vi "sq_calibrate.vi"() -> ()   [LabVIEW 2014]
uses:
  <vilib>/Analysis/6fits.llb/Curve Fitting Criteria.ctl
  <vilib>/Platform/TimedLoop/XDataNode/timing_clust.ctl
  <vilib>/Platform/TimedLoop/XDataNode/nitl_modes.ctl
  <vilib>/Platform/TimedLoop/XDataNode/wakeup.ctl
  testing/injection_point.ctl
  cancellation/decoupled_gain.ctl
  testing/probe_point.ctl
  <vilib>/Analysis/1siggen.llb/Ramp Pattern by Samples.vi
  initialization/micron_globals.vi
  <vilib>/Utility/file.llb/Write To Spreadsheet File (string).vi
  <vilib>/Analysis/polynomials.llb/1D Polynomial Evaluation (DBL).vi
  <vilib>/Platform/TimedLoop/XDataNode/XDataNode.xnode
  <vilib>/Platform/TimedLoop/XDataNode/XDNodeRunTimeDep.lvlib
  <vilib>/Analysis/NI_AALPro.lvlib
  <vilib>/Analysis/NI_AALBase.lvlib
panel:
  out "Current characteristics":string[][](table)
  in  "Order adjustment":i32[](array[numeric])=[0, 0, 0, 0, 0, 0]
  in  "Show current":bool
  in  "Show data":bool
  in  "Axis selector":bool[](array[boolean])=[TRUE, TRUE, TRUE, TRUE, TRUE, TRUE]
  out "Responses":cluster{"Ramp Pattern":dbl[], "P(A)":dbl[]}[](graph)
  in  "stop":bool
  out "Limit fail":bool
  in  "Intitialize":bool
  in  "Fit method":T1=1 items=["Least Square", "Least Absolute Residual", "Bisquare"]
  in  "Store calibration":bool
  in  "Start calibration":bool
  out "New Coefficients":dbl[][](array[numeric])
  in  "Report file":path=path "c:/test/sq_calibrate.csv"
  in  "Save report":bool
  out "Fit characteristics":string[][](table)
  in  "Dummy points":dbl[][](array[numeric])=[[-2.0, -40.0], [1.5, 25.0]]
  in  "Stimulus":T2={"Length (sec)"=2.5, "Initial amplitude"=0.05, "Frequency (Hz)"=2.0, "Nonlinearity"=5.0} {"Nonlinearity" format="%#_3p"; "Frequency (Hz)" format="%#_3p"; "Initial amplitude" format="%#_3p"; "Length (sec)" format="%#_3p"}
  out "Current Coefficients":dbl[][](array[numeric])
  in  "Offset":sgl
  in  "Amplitude":sgl=1200.0 format="%#_3p"
  in  "Fit order":i32=5
  in  "Derivitive method":u16(ring)=2 items=["2nd Order Central", "4th Order Central", "Forward", "Backward", "KF rates"]
  in  "Decimate":i32=7
  # "Motor calibration"
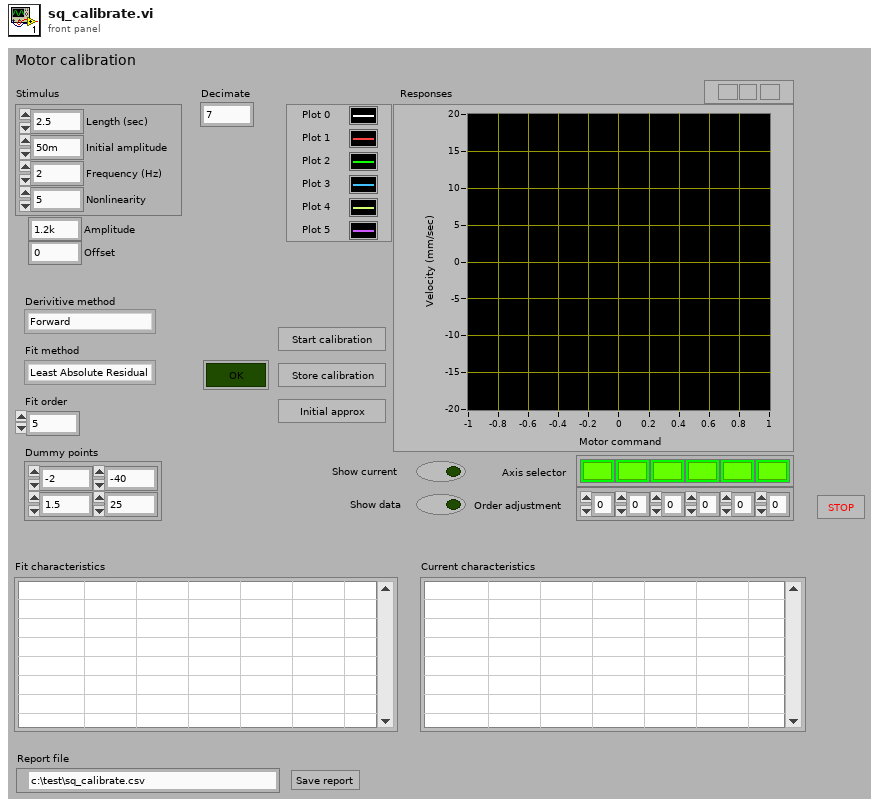
[diagram p1: front panel]
types:
  T1 = typedef "NI_AALPro.lvlib/Curve Fitting Criteria.ctl" = u16
  T2 = cluster{"Length (sec)":sgl, "Initial amplitude":sgl, "Frequency (Hz)":sgl, "Nonlinearity":sgl}
  T3 = typedef "decoupled_gain.ctl" = cluster{"XY":sgl, "Rxy":sgl, "Z":sgl, "Rz":sgl}
  T4 = typedef "injection_point.ctl" = enum16{"Total pose", "V limiter", "Goal ", "Link position", "KF link position", "Inverse kin", "Link goal", "Link error", "Controller", "Output", "Drive", "Light"}
  T5 = enum16{"Off", "Step", "Sine", "Triangle", "Arbitrary"}
  T6 = typedef "probe_point.ctl" = enum16{"Position (tip)", "Position (RCM)", "Null pos (tip)", "Null pos (RCM)", "V limiter (tip)", "V Limiter (RCM)", "Goal (tip)", "Goal (RCM)", "Link pos 0", "Link pos 1", "KF link pos 0", "KF link pos 1", "Link rate 0", "Link rate 1", "Link residue 0", "Link residue 1", "Link goal 0", "Link goal 1", "Rate limit 0", "Rate limit 1", "Link error 0", "Link error 1", "Controller 0", "Controller 1", "Output 0", "Output 1", "Drive 0", "Drive 1", "Stimulus 0", "Stimulus 1", "Trace data 0", "Trace data 1", "Analog data 0", "Analog data 1", "Status flags", "Light 0", "Light 1", "Light 2", "Light 3", "Light 4", "Light 5", "Goal origin", "Goal rotation 0", "Goal rotation 1", "Goal rotation 2", "Output origin", "Output rotation 0", "Output rotation 1", "Output rotation 2", "Handle origin", "Handle rotation 0", "Handle rotation 1", "Handle rotation 2", "Handle position", "Handle velocity", "Handle acceleration", "Handle angles", "Handle angle rates", "Handle pos residue", "Handle angle residue", "Trace length"}
  T7 = typedef "XDNodeRunTimeDep.lvlib/timing_clust.ctl" = cluster{"Expected End [f-1]":u64, "Actual End [f-1]":u64, "Finished Late? [f-1]":bool, "Expected End [i-1]":u64, "Actual End [i-1]":u64, "Finished Late? [i-1]":bool, "Expected Start [i]":u64, "Actual Start [i]":u64, "Expected Start [f]":u64, "Actual Start [f]":u64, "Source Name":string, "Structure Name":string, "Period":i64, "Deadline":i64, "Offset":i64, "Start":i64, "Priority":i32, "Timeout":i32, "Mode":T8, "Wakeup Reason":T9, "Error":errorcluster, "Source Type":string, "Secondary Source Type":string, "Global End Time":u64, "Global Start Time":u64, "Frame Duration":u64, "Iteration Duration":u64, "Assigned CPU":i32, "I/O Scan Engine Mode":u32}
  T8 = typedef "XDNodeRunTimeDep.lvlib/nitl_modes.ctl" = enum32{"No Change", "Process missed periods, maintain original phase", "Discard missed periods, maintain original phase", "Process missed periods, ignore original phase", "Discard missed periods, ignore original phase"}
  T9 = typedef "XDNodeRunTimeDep.lvlib/wakeup.ctl" = enum32{"Normal", "Aborted", "Asynchronous wakeup", "Timing source error", "Timed loop error", "Timeout"}
  T10 = typedef "Micron params.ctl" = cluster{"Stimulus":T11, "Goal Filter A":T12, "Mode controls":T13, "Manipulator type":enum16{"Current piezo", "Voltage piezo"}, "Manipulator calibration":T14, "Network":T16, "Goal Filter B":T12, "Cancellation":T17, "Transition time":sgl, "Estimation":T18}
  T11 = typedef "stimulus.ctl" = cluster{"Type":enum16{"Off", "Step", "Sine", "Triangle", "Arbitrary"}, "Phase":dbl, "Amplitude":sgl[], "Injection point":T4, "Closed loop":bool, "Offset":sgl[], "Tip -> world":bool, "Frequency":dbl, "Length":dbl}
  T12 = typedef "goal_loop_parms.ctl" = cluster{"Speedup max":sgl, "Speedup thresh":sgl, "Speedup nonlin":sgl, "Filters":cluster{"Lower Fc":sgl, "Lower Q":sgl, "Scale factor":sgl, "Upper Fc":sgl, "Upper Q":sgl, "V limit":sgl, "V limit range":sgl}[]}
  T13 = typedef "mode_conrols.ctl" = cluster{"Hold":bool, "Cancellation":bool, "Goal filter":bool, "Trigger":bool}
  T14 = typedef "manipulator_cal.ctl" = cluster{"Tool offsets":sgl[][], "Tip light calibration":T15, "Handle light calibration":T15, "Base pivots":sgl[][], "Output pivots":sgl[][], "Length center":sgl, "Workspace height":sgl[], "Workspace diameter":sgl[], "Linearization":sgl[][], "Stack travel":sgl, "Saturation pos":sgl, "Inverse filters":cluster{"filter structure":enum32{"IIR 2nd Order", "IIR 4th Order"}, "Reverse Coefficients":dbl[], "Forward Coefficients":dbl[]}[]}
  T15 = typedef "probe_calibration.ctl" = sgl[][]
  T16 = typedef "network_params.ctl" = cluster{"Remote Host":string, "Send Status":bool, "Send Port":u16, "Recv Commands":bool, "Recv Port":u16}
  T17 = typedef "sq_control_params.ctl" = cluster{"KP":T3, "KI":sgl, "KD":T3, "Max vel":sgl, "Max acc":sgl, "Int error limit":sgl, "RCM gain":sgl, "Bypass":bool, "Degraded gain":sgl}
  T18 = typedef "estimation_controls.ctl" = cluster{"Link":cluster{"Measure noise":dbl[], "Process noise":dbl[], "Alt process noise":dbl[], "Alt turnoff cycles":i32, "Innovation limit":dbl[], "Residue threshold":dbl, "Enable":bool}, "Handle":cluster{"Measure noise":dbl[], "Process noise":dbl[], "State limits":dbl[], "Innovation limit":dbl[], "Prediction Lookahead":sgl, "Enable":bool}}
  T19 = typedef "ui_override_opts.ctl" = cluster{"Triggering":bool, "Parameters":bool, "Stimulus":bool, "Calibration":bool, "Modes":bool}
  T20 = cluster{"Decimate":i32, "Derivitive method":u16, "Fit method":T1, "Fit order":i32, "Order adjustment":i32[], "Axis selector":bool[], "Show data":bool, "Show current":bool, "Dummy points":dbl[][]}
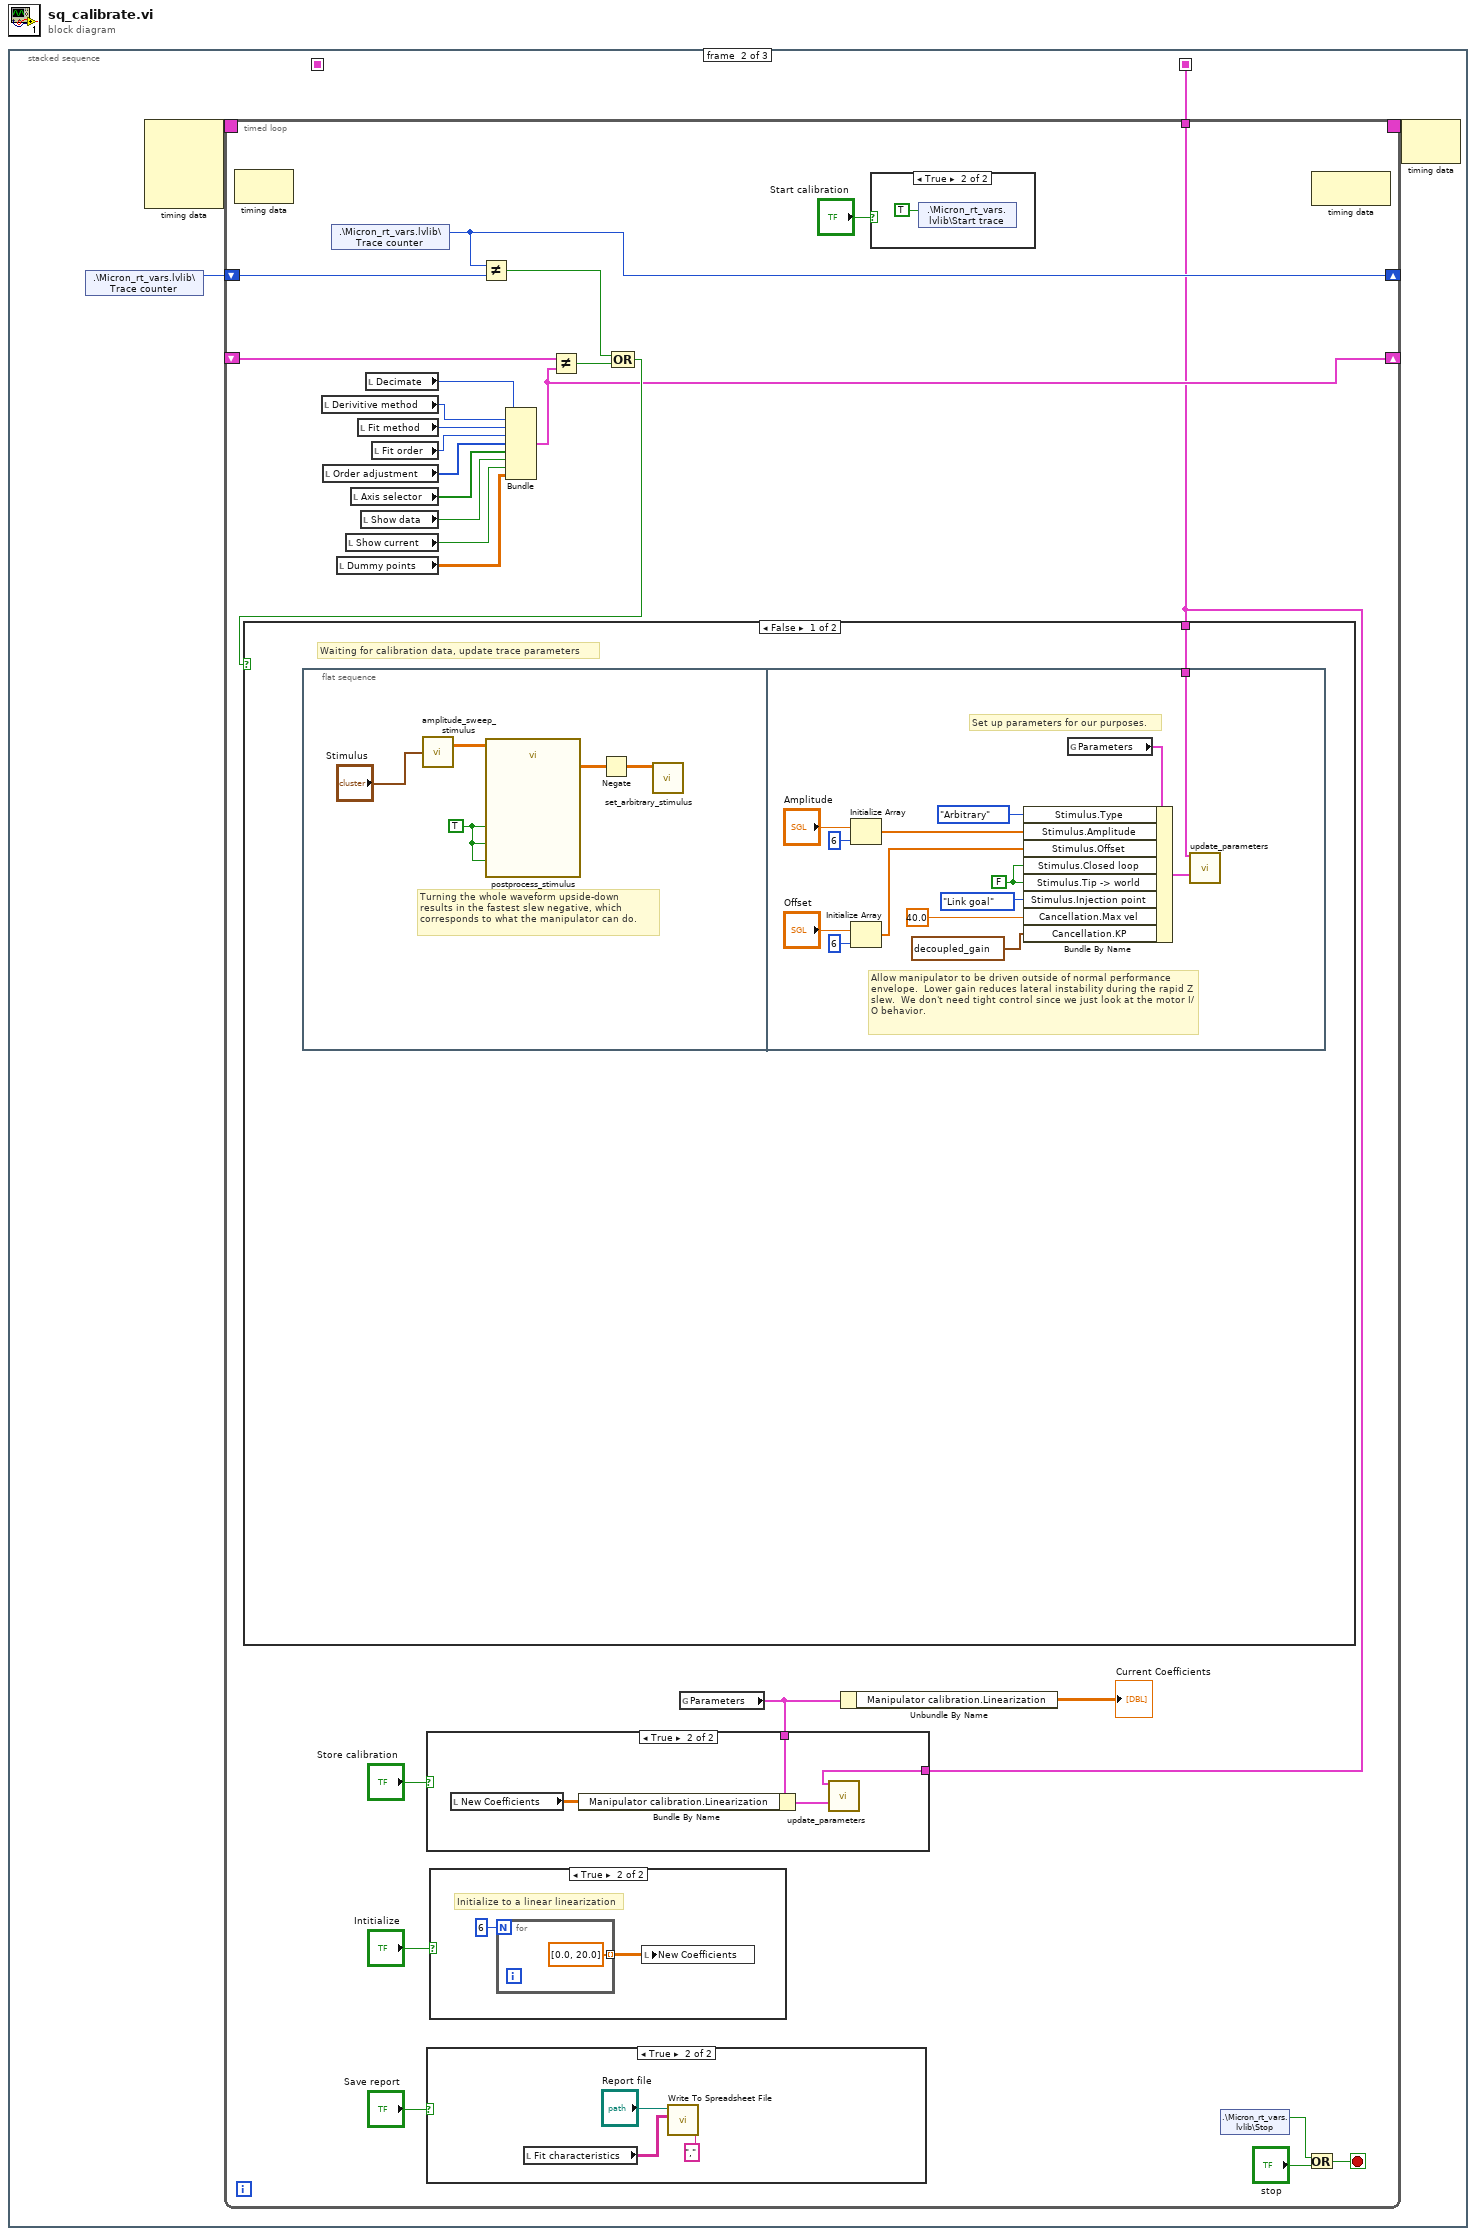
[diagram p0: block diagram]
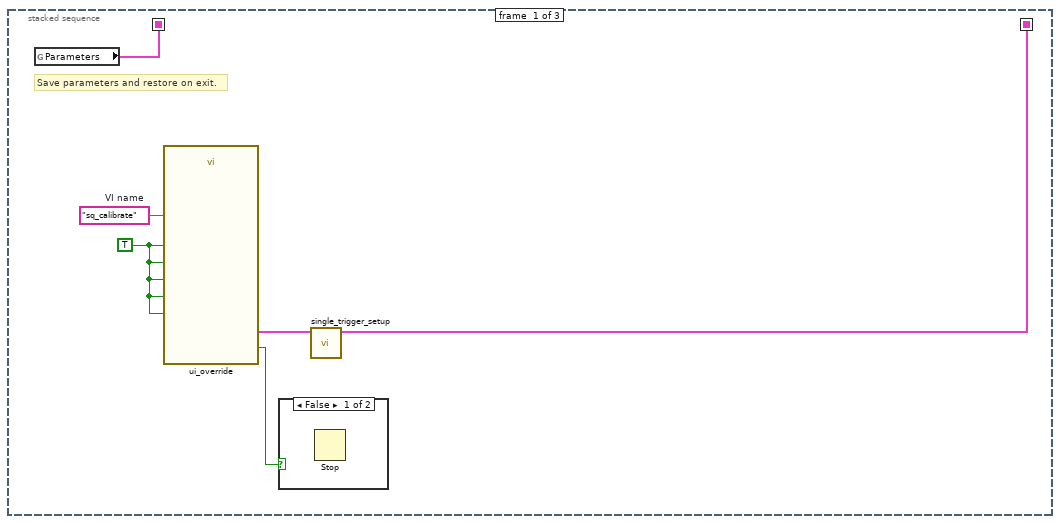
[diagram p2: hidden frame]
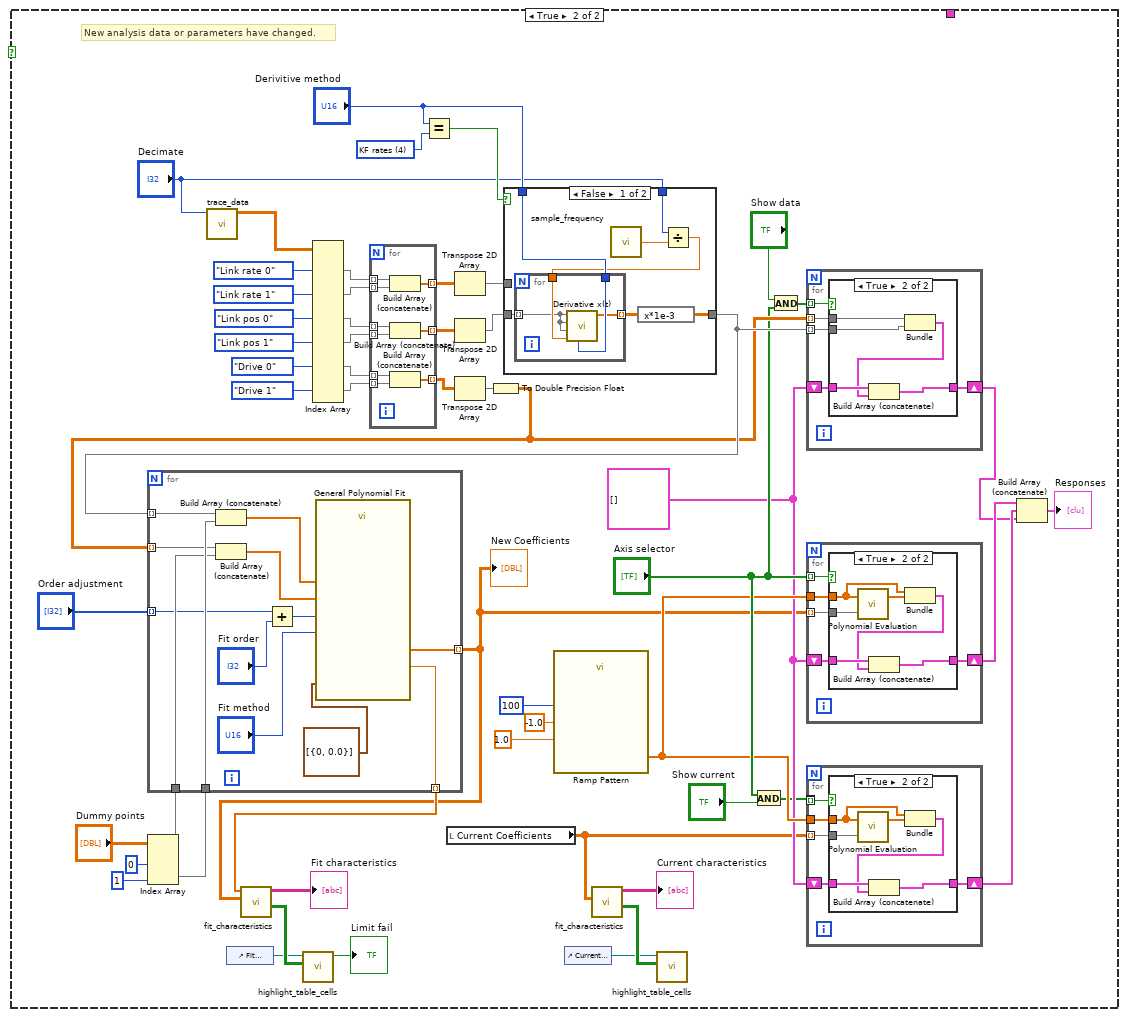
[diagram p8: hidden frame]
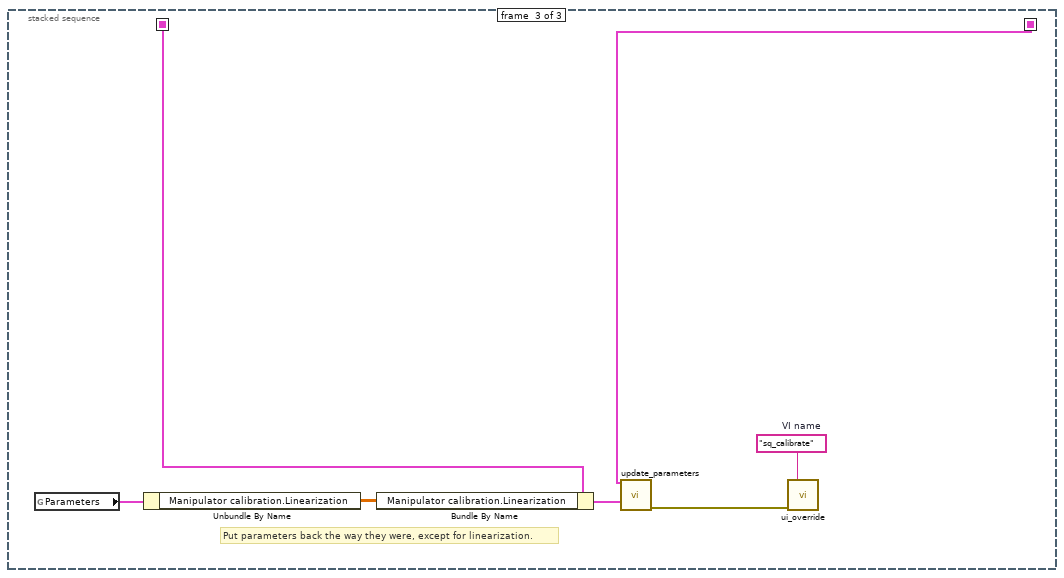
[diagram p13: hidden frame]
diagram:
  n1 = stacked-sequence {
    seq-local: [w5 _ _] -> [_ _ w200]
    seq-local: [w1 _ _] -> [_ w6 w197]
    frame #0 {
      w2 = TRUE ("All or nothing")
      w4 = "sq_calibrate"  # VI name
      # "Save parameters and restore on exit."
      n2 = global read "micron_globals.vi" "Parameters"() -> (w5:T10)
      n3 = call "ui_override.vi"("Triggering"=w2, "VI name"=w4, "Parameters"=w2, "Stimulus"=w2, "Calibration"=w2, "All or nothing"=w2) -> ("Override"=w1:T19, "Got all"=w3:bool)  [unwired: 7 in, 1 out]
      n4 = case shown="False" w3 {
        frame False {
          n5 = Stop() -> ()  [unwired: 1 in]
        }
        frame True {
        }
      }
      n6 = call "single_trigger_setup.vi"("Override in"=w1) -> ()  [unwired: 10 in, 1 out]
    }
    frame #1 {
      n7 = shared-variable ".\\Micron_rt_vars.lvlib\\Trace counter"() -> (w7:u32)  [unwired: 2 out]
      n8 = node-c288() -> (w9:T7)  [unwired: 4 out]
      n9 = timed-loop {
        timing: w9 -> [_]
        timing-out: [_] -> w8
        shift-right: [w25] -> _
        shift-left: w7 -> [w35]
        shift-right: [w22] -> _
        shift-left: _ -> [w27]
        tunnel: w6 -> [w16]
        stop <- w10 stop-if-true
        n10 = node-c288() -> ()  [unwired: 2 out]
        n11 = local read "Derivitive method"() -> (w31:u16)
        n12 = local read "Order adjustment"() -> (w28:i32[])
        n13 = shared-variable ".\\Micron_rt_vars.lvlib\\Trace counter"() -> (w25:u32)  [unwired: 2 out]
        n14 = local read "Dummy points"() -> (w15:dbl[][])
        n15 = local read "Show current"() -> (w19:bool)
        n16 = local read "Axis selector"() -> (w24:bool[])
        n17 = local read "Fit method"() -> (w30:T1)
        n18 = local read "Show data"() -> (w23:bool)
        n19 = local read "Decimate"() -> (w32:i32)
        n20 = local read "Fit order"() -> (w29:i32)
        n21 = case shown="True" "Save report" {
          frame False {
          }
          frame True {
            n22 = local read "Fit characteristics"() -> (w39:string[][])
            n23 = call-poly <vilib>:"Write To Spreadsheet File.vi"("delimiter (\\t)"="," ("delimiter (\\t)"), "2D data"=w39, "file path (dialog if empty)"="Report file") -> ()  [unwired: 5 in, 1 out]
          }
        }
        n24 = case shown="True" "Intitialize" {
          frame False {
          }
          frame True {
            # "Initialize to a linear linearization"
            n25 = for {
              N: 6 -> [_]
              tunnel: [dbl[] [0.0, 20.0]] -> w36 mode=indexing
            }
            n26 = local write "New Coefficients"(w36) -> ()
          }
        }
        n27 = Not Equal?(x=w25, y=w35) -> (x != y?=w18:bool)
        n28 = Bundle("Decimate"=w32, "Derivitive method"=w31, "Fit method"=w30, "Fit order"=w29, "Order adjustment"=w28, "Axis selector"=w24, "Show data"=w23, "Show current"=w19, "Dummy points"=w15) -> (w22:T20)  [unwired: 1 in]
        n29 = Not Equal?(x=w27, y=w22) -> (x != y?=w26:bool)
        n30 = Compound Arithmetic op=OR(w18, w26) -> (w33:bool)
        n31 = case shown="False" w33 {
          tunnel: w16 -> [w47 _]
          frame False {
            # "Waiting for calibration data, update trace parameters"
            n32 = flat-sequence {
              tunnel: w47 -> [w54]
              frame #0 {
                w50 = TRUE ("Append reversed")
                # "Turning the whole waveform upside-down\nresults in the fastest slew negative, which\ncorresponds to what the manipulator can do."
                n33 = call "amplitude_sweep_stimulus.vi"("Parameters"="Stimulus") -> ("Result"=w51:sgl[][])
                n34 = call "postprocess_stimulus.vi"("Normalize"=w50, "Negate"=w50, "Append reversed"=w50, "Input"=w51) -> ("Output"=w49:sgl[][])  [unwired: 7 in]
                n35 = Negate(x=w49) -> (-x=w48:sgl[][])
                n36 = call "set_arbitrary_stimulus.vi"("New stimulus"=w48) -> ()  [unwired: 11 in]
              }
              frame #1 {
                w60 = FALSE ("Stimulus.Closed loop")
                # "Allow manipulator to be driven outside of normal performance envelope.  Lower gain reduces lateral instability during the rapid Z slew.  We don't need tight control since we just look at the motor I/O behavior."
                # "Set up parameters for our purposes."
                n37 = Initialize Array("Amplitude", 6 ("dimension size")) -> (w61:sgl[])
                n38 = Initialize Array("Offset", 6 ("dimension size")) -> (w56:sgl[])
                n39 = global read "micron_globals.vi" "Parameters"() -> (w65:T10)
                n40 = Bundle By Name(cluster=w65, "Stimulus.Type"=T5."Arbitrary", "Stimulus.Amplitude"=w61, "Stimulus.Offset"=w56, "Stimulus.Closed loop"=w60, "Stimulus.Tip -> world"=w60, "Stimulus.Injection point"=injection_point."Link goal", "Cancellation.Max vel"=sgl 40.0, "Cancellation.KP"=T3 {"XY"=0.2, "Rxy"=0.2, "Z"=0.2, "Rz"=0.1}) -> (w66:T10)
                n41 = call "update_parameters.vi"("Modify"=w54, "Parameters"=w66) -> ()  [unwired: 12 in, 2 out]
              }
            }
          }
          frame True {
            w82 = u16 4 items=["2nd Order Central", "4th Order Central", "Forward", "Backward", "KF rates"] ("Derivitive method")
            w96 = cluster{sgl[], "dX/dt":dbl[]}[] []
            # "New analysis data or parameters have changed."
            n42 = Index Array(array="Dummy points", index (col) #1=0 ("disabled index (col)"), index (col) #2=1 ("index (col)")) -> (element #1=w88:dbl[], element #2=w89:dbl[])  [unwired: 2 in]
            n43 = call "trace_data.vi"("Decimate"="Decimate") -> ("Decimated trace"=w121:sgl[][][])  [unwired: 8 in, 2 out]
            n44 = control-ref of="Fit characteristics"() -> (w72:refnum<vi>)
            n45 = Index Array(array=w121, index (dim 1) #1=probe_point."Link rate 0" ("Probe point"), index (dim 1) #2=probe_point."Link rate 1" ("Probe point"), index (dim 1) #3=probe_point."Link pos 0" ("Probe point"), index (dim 1) #4=probe_point."Link pos 1" ("Probe point"), index (dim 1) #5=probe_point."Drive 0" ("Probe point"), index (dim 1) #6=probe_point."Drive 1" ("Probe point")) -> (element #1=w85:sgl[][], element #2=w84:sgl[][], element #3=w116:sgl[][], element #4=w115:sgl[][], element #5=w113:sgl[][], element #6=w114:sgl[][])  [unwired: 12 in]
            n46 = for {
              tunnel: w116 -> [w190] mode=indexing
              tunnel: w115 -> [w189] mode=indexing
              tunnel: w114 -> [w188] mode=indexing
              tunnel: w113 -> [w187] mode=indexing
              tunnel: [w186] -> w112 mode=indexing
              tunnel: [w185] -> w110 mode=indexing
              tunnel: w85 -> [w184] mode=indexing
              tunnel: w84 -> [w183] mode=indexing
              tunnel: [w182] -> w83 mode=indexing
              n47 = Build Array (concatenate)(w184, w183) -> (w182:sgl[])
              n48 = Build Array (concatenate)(w190, w189) -> (w186:sgl[])
              n49 = Build Array (concatenate)(w187, w188) -> (w185:sgl[])
            }
            n50 = Equal?(x="Derivitive method", y=w82) -> (x = y?=w80:bool)
            n51 = local read "Current Coefficients"() -> (w70:dbl[][])
            n52 = Transpose 2D Array(2D array=w83) -> (transposed array=w78:sgl[][])
            n53 = Transpose 2D Array(2D array=w112) -> (transposed array=w111:sgl[][])
            n54 = Transpose 2D Array(2D array=w110) -> (transposed array=w105:sgl[][])
            n55 = To Double Precision Float(number=w105) -> (double precision float=w104:dbl[][])
            n56 = case shown="False" w80 {
              tunnel: w111 -> [w128 _]
              tunnel: [w126 w133] -> w106
              tunnel: "Derivitive method" -> [w125 _]
              tunnel: "Decimate" -> [w123 _]
              tunnel: w78 -> [_ w133]
              frame False {
                n57 = call "sample_frequency.vi"() -> ("Sample frequency"=w124:dbl)
                n58 = Divide(x=w123, y=w124) -> (x/y=w122:dbl)
                n59 = for {
                  tunnel: w128 -> [w129] mode=indexing
                  tunnel: w122 -> [w132]
                  tunnel: w125 -> [w131]
                  tunnel: [w130] -> w127 mode=indexing
                  n60 = call <vilib>:"Derivative x(t).vi"("method"=w131, "dt"=w132, "Final Condition"=w129, "Initial Condition"=w129, "X"=w129) -> ("dX/dt"=w130:dbl[])  [unwired: 5 in, 1 out]
                }
                n61 = expression code="x*1e-3"(w127) -> (w126:dbl[][])
              }
              frame True {
              }
            }
            n62 = for {
              tunnel: w104 -> [w175] mode=indexing
              tunnel: w106 -> [w178] mode=indexing
              tunnel: [w180] -> w76 mode=indexing
              tunnel: [w179] -> w77 mode=indexing
              tunnel: w89 -> [w177]
              tunnel: w88 -> [w174]
              tunnel: "Order adjustment" -> [w170] mode=indexing
              n63 = Build Array (concatenate)(w178, w177) -> (w176:dbl[])
              n64 = Build Array (concatenate)(w175, w174) -> (w173:dbl[])
              n65 = Add(x=w170, y="Fit order") -> (x+y=w172:i32)
              n66 = call <vilib>:"General Polynomial Fit.vi"("Y"=w176, "polynomial order"=w172, "Coefficient Constraint"=cluster{"order":i32, "coefficient":dbl}[] [{"order"=0, "coefficient"=0.0}], "X"=w173, "method"="Fit method") -> ("Polynomial Coefficients"=w180:dbl[], "residue"=w179:dbl)  [unwired: 7 in, 2 out]
            }
            "New Coefficients" <- w76
            n67 = call "fit_characteristics.vi"("Polynomial Coefficients"=w76, "Residue"=w77) -> ("Limit fail"=w75:bool[][], "Fit characteristics"=→"Fit characteristics":string[][])  [unwired: 8 in]
            n68 = call "highlight_table_cells.vi"("Limit fail"=w75, "Table in"=w72) -> ("Some limit fail"=→"Limit fail":bool)  [unwired: 9 in]
            n69 = call-poly <vilib>:"Ramp Pattern.vi"("start"=-1.0, "end"=1.0, "samples"=100) -> ("Ramp Pattern"=w97:dbl[])  [unwired: 7 in, 1 out]
            n70 = control-ref of="Current characteristics"() -> (w67:refnum<vi>)
            n71 = call "fit_characteristics.vi"("Polynomial Coefficients"=w70) -> ("Limit fail"=w68:bool[][], "Fit characteristics"=→"Current characteristics":string[][])  [unwired: 9 in]
            n72 = call "highlight_table_cells.vi"("Limit fail"=w68, "Table in"=w67) -> ()  [unwired: 9 in, 1 out]
            n73 = And(x="Axis selector", y="Show current") -> (x .and. y?=w95:bool[])
            n74 = And(x="Show data", y="Axis selector") -> (x .and. y?=w101:bool[])
            n75 = for {
              tunnel: w101 -> [w150] mode=indexing
              shift-right: [w148] -> w93
              shift-left: w96 -> [w149]
              tunnel: w104 -> [w147] mode=indexing
              tunnel: w106 -> [w146] mode=indexing
              n76 = case shown="True" w150 {
                tunnel: w149 -> [w151 w156]
                tunnel: [w151 w154] -> w148
                tunnel: w147 -> [_ w153]
                tunnel: w146 -> [_ w152]
                frame False {
                }
                frame True {
                  n77 = Bundle(w153, "dX/dt"=w152) -> (w155:cluster{dbl[], "dX/dt":dbl[]})  [unwired: 1 in]
                  n78 = Build Array (concatenate)(w156, w155) -> (w154:cluster{dbl[], "dX/dt":dbl[]}[])
                }
              }
            }
            n79 = for {
              tunnel: w97 -> [w161]
              tunnel: w76 -> [w160] mode=indexing
              tunnel: "Axis selector" -> [w159] mode=indexing
              shift-right: [w157] -> w103
              shift-left: w96 -> [w158]
              n80 = case shown="True" w159 {
                tunnel: w161 -> [_ w165]
                tunnel: w160 -> [_ w168]
                tunnel: w158 -> [w162 w167]
                tunnel: [w162 w163] -> w157
                frame False {
                }
                frame True {
                  n81 = call-poly <vilib>:"Polynomial Evaluation.vi"("P(x)"=w168, "A"=w165) -> ("P(A)"=w166:dbl[])  [unwired: 1 out]
                  n82 = Bundle("Ramp Pattern"=w165, "P(A)"=w166) -> (w164:cluster{"Ramp Pattern":dbl[], "P(A)":dbl[]})  [unwired: 1 in]
                  n83 = Build Array (concatenate)(w167, w164) -> (w163:cluster{"Ramp Pattern":dbl[], "P(A)":dbl[]}[])
                }
              }
            }
            n84 = for {
              tunnel: w97 -> [w138]
              tunnel: w70 -> [w137] mode=indexing
              tunnel: [w134] -> _ mode=indexing
              shift-right: [w135] -> w94
              shift-left: w96 -> [w136]
              tunnel: w95 -> [w134] mode=indexing
              n85 = case shown="True" w134 {
                tunnel: w138 -> [_ w142]
                tunnel: w137 -> [_ w145]
                tunnel: w136 -> [w139 w144]
                tunnel: [w139 w140] -> w135
                frame False {
                }
                frame True {
                  n86 = call-poly <vilib>:"Polynomial Evaluation.vi"("P(x)"=w145, "A"=w142) -> ("P(A)"=w143:dbl[])  [unwired: 1 out]
                  n87 = Bundle("Ramp Pattern"=w142, "P(A)"=w143) -> (w141:cluster{"Ramp Pattern":dbl[], "P(A)":dbl[]})  [unwired: 1 in]
                  n88 = Build Array (concatenate)(w144, w141) -> (w140:cluster{"Ramp Pattern":dbl[], "P(A)":dbl[]}[])
                }
              }
            }
            n89 = Build Array (concatenate)(w103, w94, w93) -> (→"Responses":cluster{"Ramp Pattern":dbl[], "dX/dt":dbl[]}[])
          }
        }
        n90 = global read "micron_globals.vi" "Parameters"() -> (w21:T10)
        n91 = case shown="True" "Store calibration" {
          tunnel: w21 -> [_ w46]
          tunnel: w16 -> [_ w43]
          frame False {
          }
          frame True {
            n92 = local read "New Coefficients"() -> (w44:dbl[][])
            n93 = Bundle By Name(cluster=w46, "Manipulator calibration.Linearization"=w44) -> (w45:T10)
            n94 = call "update_parameters.vi"("Modify"=w43, "Parameters"=w45) -> ()  [unwired: 12 in, 2 out]
          }
        }
        n95 = Unbundle By Name(w21) -> ("Manipulator calibration.Linearization"=→"Current Coefficients":sgl[][])
        n96 = case shown="True" "Start calibration" {
          frame False {
          }
          frame True {
            n97 = shared-variable ".\\Micron_rt_vars.lvlib\\Start trace"(TRUE ("Start trace")) -> ()  [unwired: 2 out]
          }
        }
        n98 = shared-variable ".\\Micron_rt_vars.lvlib\\Stop"() -> (w12:bool)  [unwired: 2 out]
        n99 = Or(x=w12, y="stop") -> (x .or. y?=w10:bool)
        n100 = node-c288() -> ()  [unwired: 2 out]
      }
      n101 = node-c288(w8) -> ()  [unwired: 1 out]
    }
    frame #2 {
      w196 = "sq_calibrate"  # VI name
      # "Put parameters back the way they were, except for linearization."
      n102 = global read "micron_globals.vi" "Parameters"() -> (w201:T10)
      n103 = Unbundle By Name(w201) -> ("Manipulator calibration.Linearization"=w199:sgl[][])
      n104 = Bundle By Name(cluster=w200, "Manipulator calibration.Linearization"=w199) -> (w198:T10)
      n105 = call "update_parameters.vi"("Modify"=w197, "Parameters"=w198) -> ("error out"=w195:errorcluster)  [unwired: 12 in, 1 out]
      n106 = call "ui_override.vi"("VI name"=w196, "error in"=w195) -> ()  [unwired: 11 in, 3 out]
    }
  }
